vi "GetGraphScaleReference.vi"(8 "error in":errorcluster, 11 "GraphScale in":refnum<class "GraphScale.lvclass">) -> (0 "error out":errorcluster, 1 "graph scale reference":refnum<vi>, 3 "GraphScale out":refnum<class "GraphScale.lvclass">)   [LabVIEW 2014, in "Raspberry Pi Compatible Compiler for LabVIEW.lvlib" / "GraphScale.lvclass"]
uses:
  GraphScale.lvclass
  Generic/Generic.lvclass
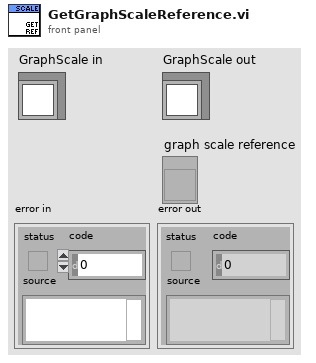
[diagram p1: front panel]
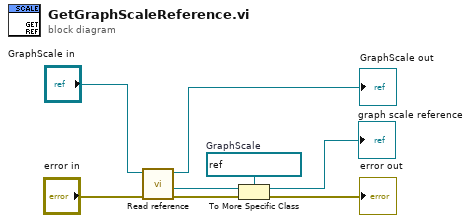
[diagram p0: block diagram]
diagram:
  w5 = refnum<vi> refnum  # GraphScale
  n1 = call "Read reference.vi"("error in"="error in", "GObject in"="GraphScale in") -> ("error out"=w6:errorcluster, "reference"=w7:refnum<vi>, "GObject out"=→"GraphScale out":refnum<class "GraphScale.lvclass">)  [unwired: 5 in]
  n2 = To More Specific Class(target class=w5, reference=w7, error in=w6) -> (specific class reference=→"graph scale reference":refnum<vi>, error out=→"error out":errorcluster)
